vi "Get Source Function.vi"(8 "error in (no error)":errorcluster, 11 "VISA resource name":refnum<visa-resource-name>) -> (0 "error out":errorcluster, 2 "Source Function":string, 3 "VISA resource name out":refnum<visa-resource-name>)   [LabVIEW 2024, in "Keithley 2450.lvlib"]
doc: "Gets the source function on the instrument."
uses:
  Keithley 2450.lvlib
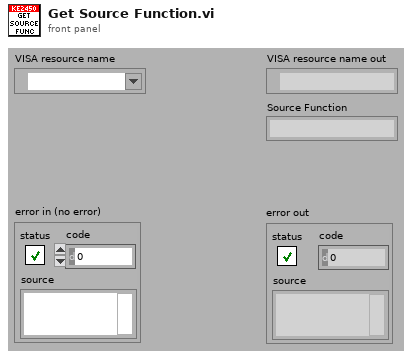
[diagram p1: front panel]
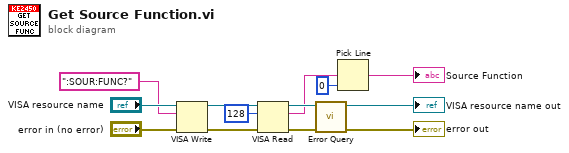
[diagram p0: block diagram]
diagram:
  n1 = VISA Write(VISA resource name="VISA resource name", write buffer=":SOUR:FUNC?", error in (no error)="error in (no error)") -> (VISA resource name out=w6:refnum<visa-resource-name>, error out=w8:errorcluster)  [unwired: 1 out]
  n2 = VISA Read(VISA resource name=w6, byte count=u32 128, error in (no error)=w8) -> (VISA resource name out=w5:refnum<visa-resource-name>, read buffer=w3:string, error out=w7:errorcluster)  [unwired: 1 out]
  n3 = call "Error Query.vi"("error in (no error)"=w7, "VISA resource name"=w5) -> ("error out"=→"error out":errorcluster, "VISA resource name out"=→"VISA resource name out":refnum<visa-resource-name>)  [unwired: 8 out]
  n4 = Pick Line(multi-line string=w3, line index=0) -> (output string=→"Source Function":string)  [unwired: 1 in]
